vi "GIBBSdll.vi"(8 "error in (no error)":errorcluster, 9 "z":dbl[](array[numeric]), 10 "D":dbl, 11 "t":dbl) -> (0 "error out":errorcluster, 2 "Ar":dbl, 3 "Gr":dbl)   [LabVIEW 2016]
doc: "subroutine GIBBSdll(t, d, z, ar, gr)\nCompute residual Helmholtz and Gibbs energies as functions of temperature, density, and composition from core functions, calculated as: \n\nG(T,D) - G0(T,P*) = G(T,D) - G0(T,D) + RTln(RTD/P*)\n\nWhere G0 is the ideal-gas state and P* is a reference pressure that is equal to the current pressure of interest. Since Gr is used only as a difference in phase equilibria calculations where the temperature and pressure of the phases are equal, the (RT/P*) part of the log term will cancel and is omitted.\n\nNormal (not residual) A and G are computed by subroutine AG.\n\nSee warning in suroutines THERM or ALLPROPS.\n\nBased on derivations in Younglove & McLinden, JPCRD 23 #5, 1994,\nequations A8 - A12\n\nINPUTS:\nt -- Temperature [K]\nd -- Molar density [mol/L]\nz -- Composition (array of mole fractions)\n\nOUTPUTS:\nar -- Residual Helmholtz energy [J/mol]\ngr -- Residual Gibbs free energy [J/mol]"
uses:
  REFPROP.DLL
panel:
  # "REFPROP-GIBBSdll.vi"
  # "void  GIBBSdll(double *t, double *D, double *z, double *ar, double *gr)"
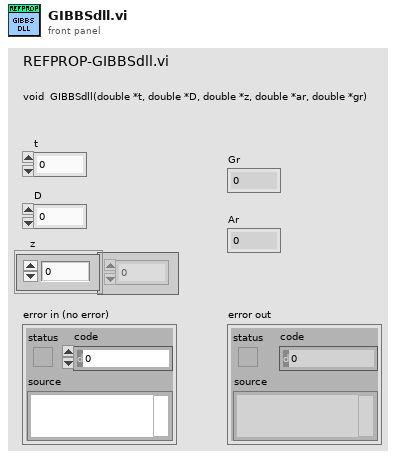
[diagram p1: front panel]
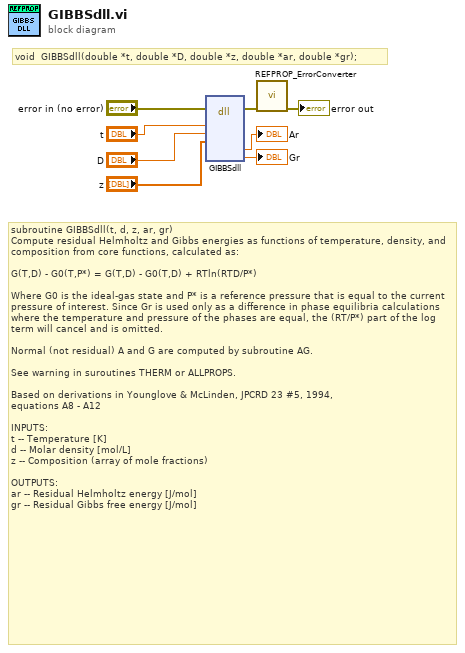
[diagram p0: block diagram]
diagram:
  # "void  GIBBSdll(double *t, double *D, double *z, double *ar, double *gr);"
  # "subroutine GIBBSdll(t, d, z, ar, gr)\nCompute residual Helmholtz and Gibbs energies as functions of temperature, density, and composition from core functions, calculated as: \n\nG(T,D) - G0(T,P*) = G(T,D) - G0(T,D) + RTln(RTD/P*)\n\nWhere G0 is the ideal-gas state and P* is a reference pressure that is equal to the current pressure of interest. Since Gr is used only as a difference in phase equilibria calculations where the temperature and pressure of the phases are equal, the (RT/P*) part of the log term will cancel and is omitted.\n\nNormal (not residual) A and G are computed by subroutine AG.\n\nSee warning in suroutines THERM or ALLPROPS.\n\nBased on derivations in Younglove & McLinden, JPCRD 23 #5, 1994,\nequations A8 - A12\n\nINPUTS:\nt -- Temperature [K]\nd -- Molar density [mol/L]\nz -- Composition (array of mole fractions)\n\nOUTPUTS:\nar -- Residual Helmholtz energy [J/mol]\ngr -- Residual Gibbs free energy [J/mol]"
  n1 = dll-call lib="S:/009 - Testing/02 - Performance Testing/REFPROP/REFPROP.*" fn="GIBBSdll"(error in="error in (no error)", "t"="t", "D"="D", "z"="z") -> (error out=w3:errorcluster, "ar"=→"Ar":dbl, "gr"=→"Gr":dbl)  [unwired: 8 in, 1 out]
  n2 = call "REFPROP_ErrorConverter.vi"("error in (no error)"=w3) -> ("error out"=→"error out":errorcluster)  [unwired: 10 in]
